vi "TCP_write.vi"(2 "error in (no error)":errorcluster, 3 "Data to send":string, 4 "Parameter to Server":string, 5 "TCP ID in":refnum<k5>) -> (0 "error out (no error)":errorcluster, 1 "TCP ID out":refnum<k5>)   [LabVIEW 2011]
doc: "Sends the data to the client"
panel:
  in  "timeout ms (2000)":i32=2000
  out "Bytes Written":i32
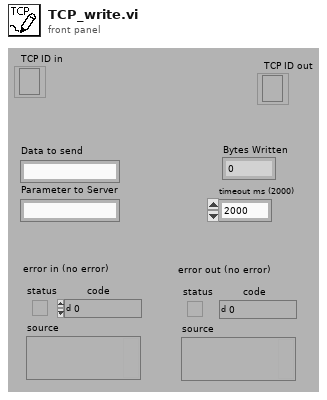
[diagram p1: front panel]
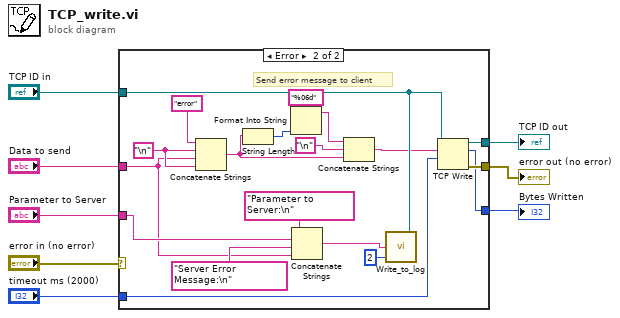
[diagram p0: block diagram]
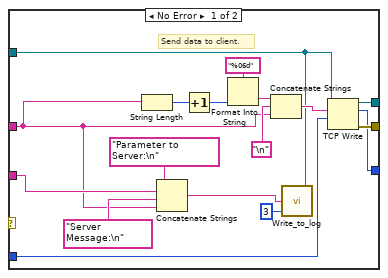
[diagram p2: hidden frame]
diagram:
  n1 = case shown="Error" "error in (no error)" {
    tunnel: "Data to send" -> [w11 w31]
    tunnel: "TCP ID in" -> [w15 w34]
    tunnel: [w22 w43] -> w5
    tunnel: [w21 w42] -> w8
    tunnel: "timeout ms (2000)" -> [w20 w41]
    tunnel: [w18 w38] -> w3
    tunnel: "Parameter to Server" -> [w12 w32]
    frame No Error {
      # "Send data to client."
      n2 = String Length(string=w11) -> (length=w10:i32)
      n3 = Concatenate Strings("Parameter to Server:\n" ("string"), w12, "Server Message:\n" ("string"), w11) -> (w14:string)
      n4 = Increment(x=w10) -> (x+1=w9:i32)
      n5 = Format Into String(format string="%06d" ("Format String"), w9) -> (resulting string=w25:string)  [unwired: 2 in, 1 out]
      n6 = Concatenate Strings(w25, "\n" ("string"), w11) -> (w23:string)
      n7 = call "Write_to_log.vi"("TCP Refnum"=w15, "Type"=i8 3, "Message"=w14) -> ()  [unwired: 1 in]
      n8 = TCP Write(connection ID=w15, data in=w23, 9:w20) -> (connection ID out=w22:refnum<k5>, bytes written=w18:i32, error out=w21:errorcluster)  [unwired: 1 in]
    }
    frame Error {
      w39 = "\n"
      # "Send error message to client"
      n9 = Concatenate Strings("error", w39, w31, w39) -> (w28:string)
      n10 = String Length(string=w28) -> (length=w30:i32)
      n11 = Format Into String(format string="%06d" ("Format String"), w30) -> (resulting string=w29:string)  [unwired: 2 in, 1 out]
      n12 = Concatenate Strings("Parameter to Server:\n" ("string"), w32, "Server Error Message:\n" ("string"), w31) -> (w33:string)
      n13 = Concatenate Strings(w29, "\n", w28) -> (w27:string)
      n14 = call "Write_to_log.vi"("TCP Refnum"=w34, "Type"=i8 2, "Message"=w33) -> ()  [unwired: 1 in]
      n15 = TCP Write(connection ID=w34, data in=w27, 9:w41) -> (connection ID out=w43:refnum<k5>, bytes written=w38:i32, error out=w42:errorcluster)  [unwired: 1 in]
    }
  }
  "error out (no error)" <- w8
  "TCP ID out" <- w5
  "Bytes Written" <- w3
